vi "sinanju_stepy.vi"(5 "错误输入（无错误）":errorcluster, 6 "t":sgl=1.0, 7 "d":sgl=20.0, 8 "mode":i32, 9 "page":i32, 10 "ax":i32, 11 "VISA资源名称":refnum<visa-resource-name>) -> (2 "错误输出":errorcluster, 3 "VISA资源名称输出":refnum<visa-resource-name>)   [LabVIEW 2017]
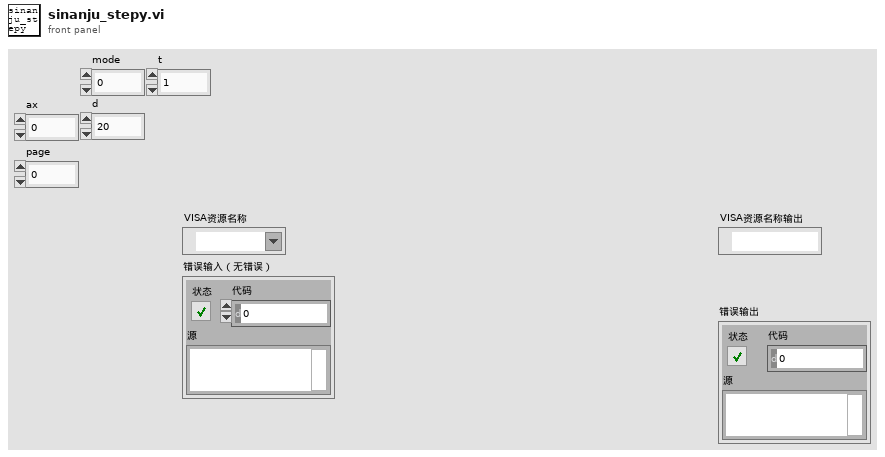
[diagram p1: front panel]
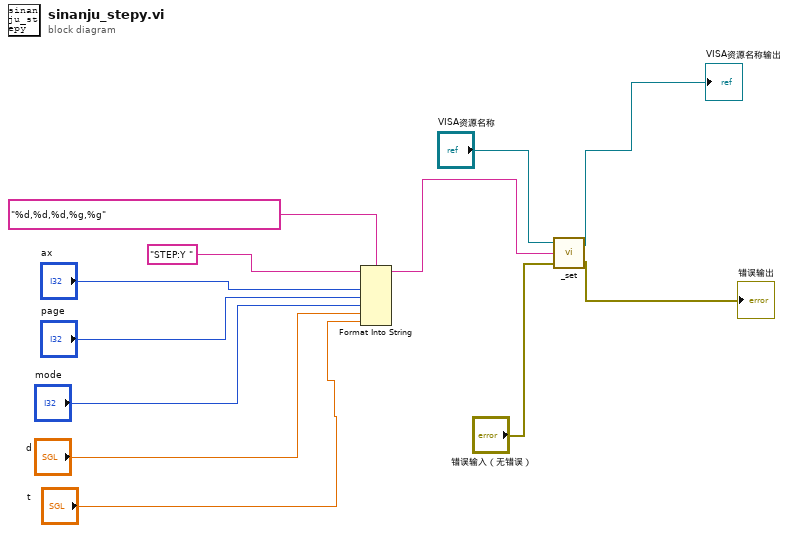
[diagram p0: block diagram]
diagram:
  n1 = Format Into String(format string="%d,%d,%d,%g,%g" ("格式字符串"), initial string="STEP:Y " ("初始字符串"), "ax", "page", "mode", "d", "t") -> (resulting string=w7:string)  [unwired: 1 in, 1 out]
  n2 = call "_set.vi"("错误输入（无错误）"="错误输入（无错误）", "写入缓冲区"=w7, "VISA资源名称输出 2"="VISA资源名称") -> ("错误输出"=→"错误输出":errorcluster, "VISA资源名称输出"=→"VISA资源名称输出":refnum<visa-resource-name>)
